vi "Delay.vi"(1 "Timer Going?":bool, 2 "Time to Wait (ms)":dbl) -> (0 "Time Up":bool)   [LabVIEW 2013]
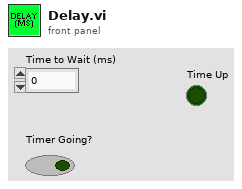
[diagram p1: front panel]
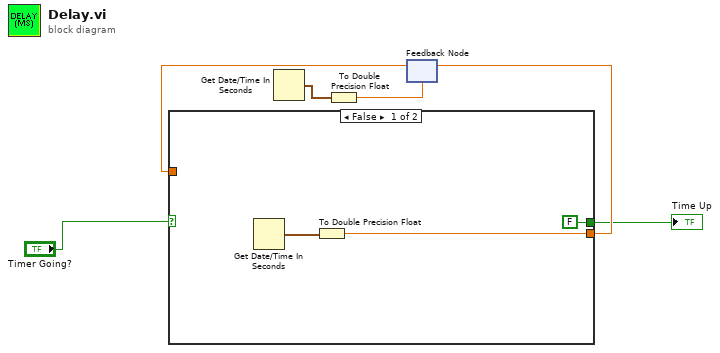
[diagram p0: block diagram]
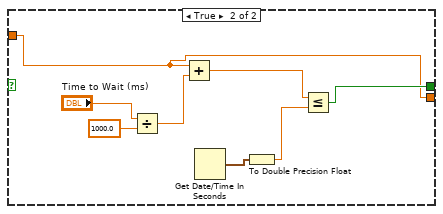
[diagram p2: hidden frame]
diagram:
  n1 = Get Date/Time In Seconds() -> (seconds since 1Jan1904=w2:timestamp)
  n2 = To Double Precision Float(number=w2) -> (double precision float=w1:dbl)
  n3 = feedback #1(w1) -> (w4:dbl)
  n4 = case shown="False" "Timer Going?" {
    tunnel: [w8 w10] -> w5
    tunnel: w4 -> [_ w10]
    tunnel: [FALSE w11] -> w3
    frame False {
      n5 = Get Date/Time In Seconds() -> (seconds since 1Jan1904=w9:timestamp)
      n6 = To Double Precision Float(number=w9) -> (double precision float=w8:dbl)
    }
    frame True {
      n7 = Divide(x="Time to Wait (ms)", y=1000.0) -> (x/y=w15:dbl)
      n8 = Add(x=w10, y=w15) -> (x+y=w13:dbl)
      n9 = Get Date/Time In Seconds() -> (seconds since 1Jan1904=w14:timestamp)
      n10 = To Double Precision Float(number=w14) -> (double precision float=w12:dbl)
      n11 = Less Or Equal?(x=w13, y=w12) -> (x <= y?=w11:bool)
    }
  }
  "Time Up" <- w3
  n12 = feedback-in #1(w5) -> ()
